vi "Draw Legend Cluster.vi"(8 "error in (no error)":errorcluster, 9 "Plot Area Ref":refnum<vi>, 10 "Number Of Rows":i32, 11 "2D Plot in":refnum<class "2D Plot.lvclass">) -> (0 "error out":errorcluster, 1 "Legend Cluster":T1(array[cluster]), 3 "2D Plot out":refnum<class "2D Plot.lvclass">)   [LabVIEW 2020, in "2D Plot.lvclass"]
uses:
  <vilib>/Math Plots/2D Math Plots/2D Plot/2D Plot/2D Plot.lvclass
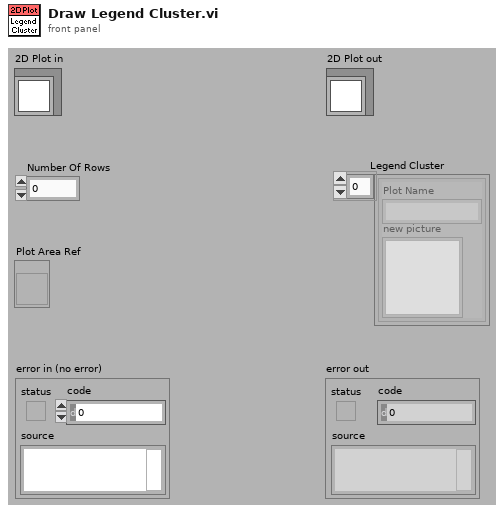
[diagram p1: front panel]
types:
  T1 = cluster{"Plot Name":string, "new picture":picture}[]
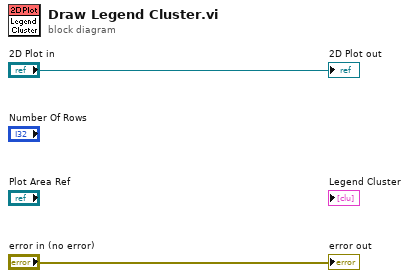
[diagram p0: block diagram]
diagram:
  "2D Plot out" <- "2D Plot in"
  "error out" <- "error in (no error)"
